vi "FGV_saltos.vi"(7 "action":enum16{"suma", "resta", "set_start", "get"}(ring)=enum."set_start", 8 "error in (no error)":errorcluster, 9 "NivRef in in":dbl, 11 "valor del salto":dbl) -> (0 "error out":errorcluster, 1 "NivRef out":dbl)   [LabVIEW 2019, in "Prueba10.lvclass"]
uses:
  Prueba10.lvclass
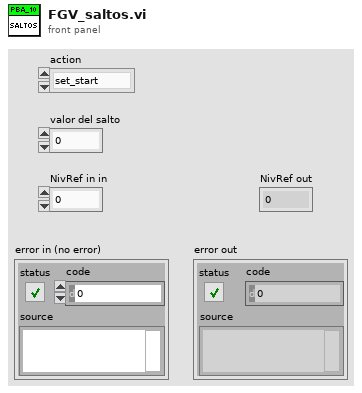
[diagram p1: front panel]
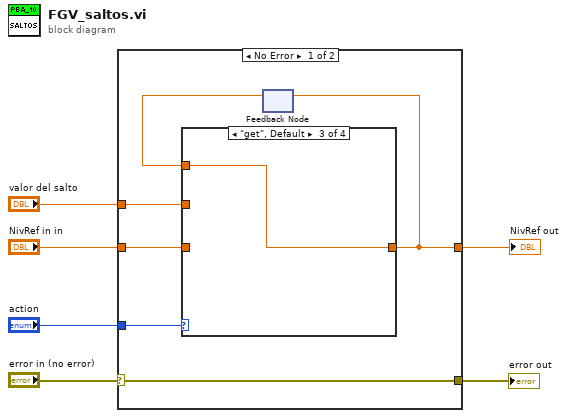
[diagram p0: block diagram]
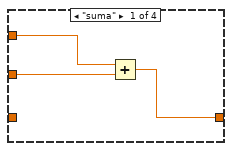
[diagram p2: hidden frame]
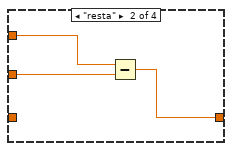
[diagram p3: hidden frame]
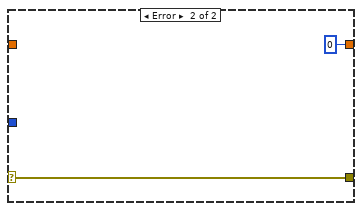
[diagram p5: hidden frame]
diagram:
  n1 = case shown="No Error" "error in (no error)" {
    selector: "error in (no error)" -> [w8 w22]
    tunnel: "action" -> [w12 _]
    tunnel: [w10 0 ("fila_inicial")] -> w5
    tunnel: "NivRef in in" -> [w9 _]
    tunnel: [w8 w22] -> w2
    tunnel: "valor del salto" -> [w7 _]
    frame No Error {
      n2 = feedback #1() -> (w11:dbl)  [unwired: 1 in]
      n3 = case shown="\"get\", Default" w12 {
        tunnel: w11 -> [w13 w16 w19 _]
        tunnel: [w14 w17 w19 w20] -> w10
        tunnel: w9 -> [_ _ _ w20]
        tunnel: w7 -> [w15 w18 _ _]
        frame "suma" {
          n4 = Add(x=w13, y=w15) -> (x+y=w14:dbl)
        }
        frame "resta" {
          n5 = Subtract(x=w16, y=w18) -> (x-y=w17:dbl)
        }
        frame "get", Default {
        }
        frame "set_start" {
        }
      }
      n6 = feedback-in #1(w10) -> ()
    }
    frame Error {
    }
  }
  "NivRef out" <- w5
  "error out" <- w2
